vi "Process Listbox.vi"(10 "Select":i32, 11 "Item Symbols in":i32[](array[numeric])) -> (3 "Item Symbols out":i32[](array[numeric]))   [LabVIEW 2019, in "Electronic Load.lvlib" / "Electronic Load.lvclass"]
uses:
  Library/Electronic Load.lvclass
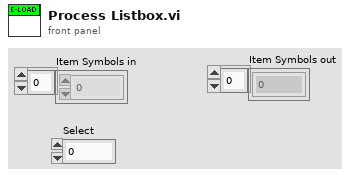
[diagram p1: front panel]
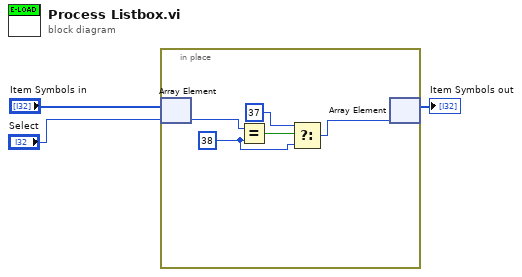
[diagram p0: block diagram]
diagram:
  n1 = in-place {
    w5 = 38
    n2 = in-place-array #1("Item Symbols in", "Select") -> (w7:i32)
    n3 = Equal?(x=w7, y=w5) -> (x = y?=w8:bool)
    n4 = Select(t=37, s=w8, f=w5) -> (s? t:f=w4:i32)
    n5 = in-place-array #1(w4) -> (→"Item Symbols out":i32[])  [unwired: 1 out]
  }
